vi "Centre Target.vi"(0 "Focus and Tracking":T4, 1 "Calibration":T5, 2 "System of Reference Interface":T3, 3 "Target":T2, 5 "error in (no error)":errorcluster, 9 "Refocus threshold":dbl=0.125) -> (13 "CFS":dbl, 14 "Target Coordinates [um]":T1, 15 "Optical Coordinates [um]":cluster{"X":dbl, "Y":dbl, "Z":dbl}, 16 "Need to refocus":bool, 17 "Scope Error":bool, 18 "Target OK":bool, 19 "error out":errorcluster)   [LabVIEW 2012, in "Targeting Unit.lvlib"]
uses:
  Targeting Unit.lvlib
  <vilib>/Analysis/Matrix/Datatypes/RealMatrix.ctl
  <vilib>/Analysis/Matrix/NI_Matrix.lvlib
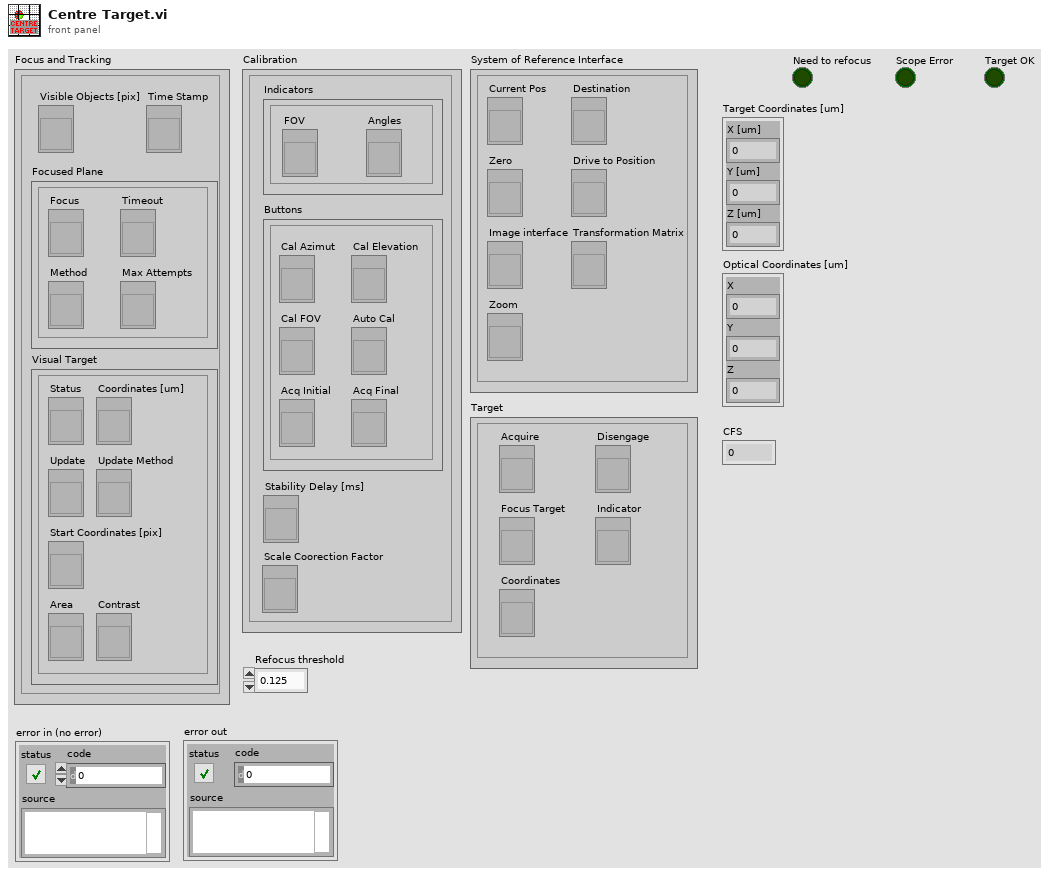
[diagram p1: front panel]
types:
  T1 = cluster{"X [um]":dbl, "Y [um]":dbl, "Z [um]":dbl}
  T2 = cluster{"Coordinates":refnum<vi>, "Acquire":refnum<vi>, "Disengage":refnum<vi>, "Indicator":refnum<vi>, "Focus Target":refnum<vi>}
  T3 = cluster{"Current Pos":refnum<vi>, "Image interface":refnum<vi>, "Transformation Matrix":refnum<vi>, "Zero":refnum<vi>, "Destination":refnum<vi>, "Drive to Position":refnum<vi>, "Zoom":refnum<vi>}
  T4 = cluster{"Focused Plane":cluster{"Focus":refnum<vi>, "Timeout":refnum<vi>, "Max Attempts":refnum<vi>, "Method":refnum<vi>}, "Time Stamp":refnum<vi>, "Visual Target":cluster{"Coordinates [um]":refnum<vi>, "Status":refnum<vi>, "Update":refnum<vi>, "Update Method":refnum<vi>, "Start Coordinates [pix]":refnum<vi>, "Area":refnum<vi>, "Contrast":refnum<vi>}, "Visible Objects [pix]":refnum<vi>}
  T5 = cluster{"Indicators":cluster{"FOV":refnum<vi>, "Angles":refnum<vi>}, "Buttons":cluster{"Cal FOV":refnum<vi>, "Cal Azimut":refnum<vi>, "Cal Elevation":refnum<vi>, "Auto Cal":refnum<vi>, "Acq Initial":refnum<vi>, "Acq Final":refnum<vi>}, "Stability Delay [ms]":refnum<vi>, "Scale Coorection Factor":refnum<vi>}
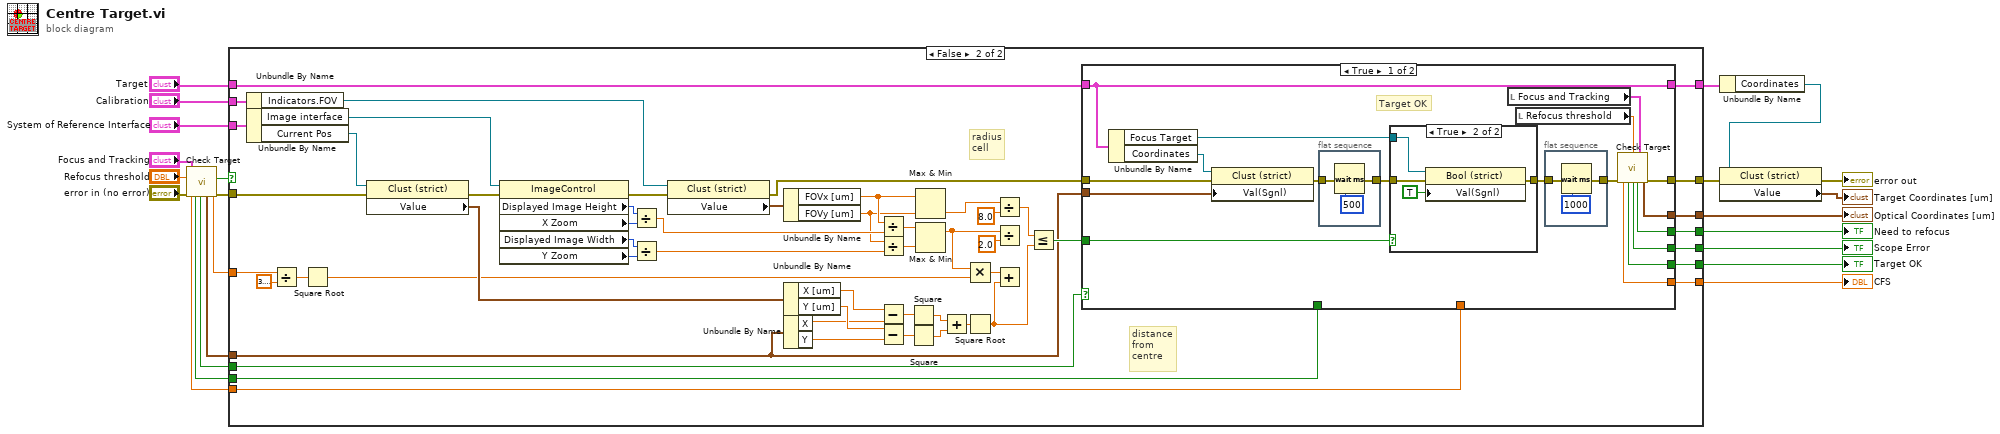
[diagram p0: block diagram]
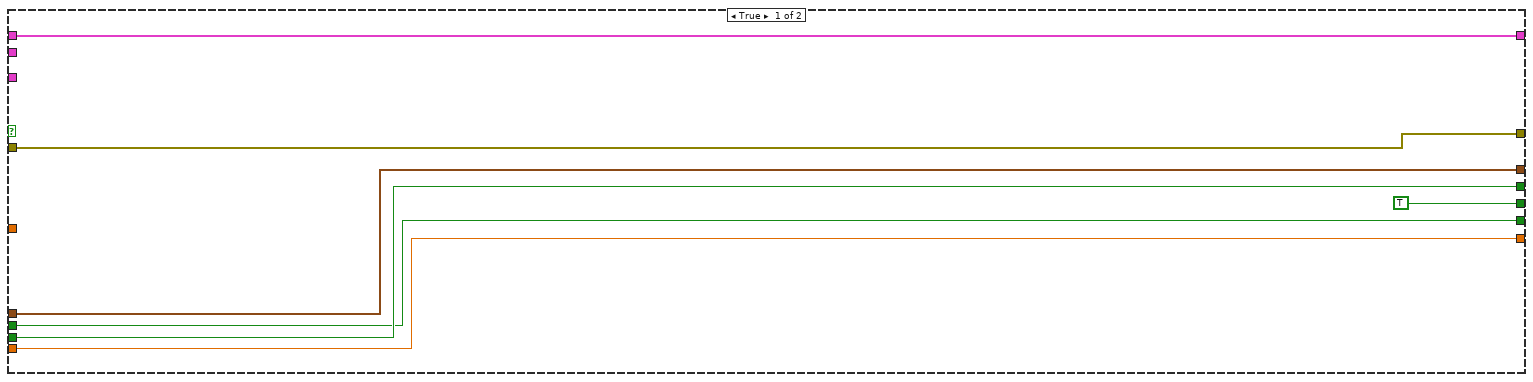
[diagram p2: hidden frame]
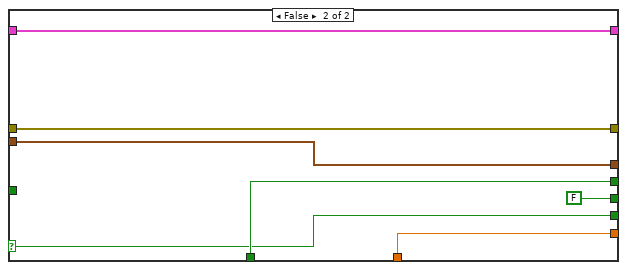
[diagram p4: hidden frame]
diagram:
  n1 = call "Check Target.vi"("Error In"="error in (no error)", "Refocus threshold"="Refocus threshold", "Focus and Tracking"="Focus and Tracking") -> ("Error out"=w16:errorcluster, "CFS"=w6:dbl, "Scope Error"=w14:bool, "Target OK"=w2:bool, "Optical Coordinates [um]"=w12:cluster{"X":dbl, "Y":dbl, "Z":dbl}, "Need to refocus"=w5:bool, "Area"=w1:dbl)  [unwired: 2 in]
  n2 = case shown="False" w14 {
    tunnel: "Calibration" -> [_ w74]
    tunnel: "System of Reference Interface" -> [_ w73]
    tunnel: [w27 w58] -> w20
    tunnel: w16 -> [w27 w43]
    tunnel: [TRUE ("Error") w50] -> w21
    tunnel: w12 -> [w29 w45]
    tunnel: "Target" -> [w28 w56]
    tunnel: [w29 w54] -> w9
    tunnel: [w28 w55] -> w8
    tunnel: [w25 w53] -> w7
    tunnel: w6 -> [w26 w52]
    tunnel: w5 -> [w25 w51]
    tunnel: [w24 w49] -> w3
    tunnel: [w26 w48] -> w4
    tunnel: w2 -> [w24 w47]
    tunnel: w1 -> [_ w44]
    frame True {
    }
    frame False {
      # "distance\nfrom\ncentre"
      # "radius\ncell"
      n3 = Unbundle By Name(w74) -> ("Indicators.FOV"=w75:refnum<vi>)
      n4 = Unbundle By Name(w73) -> ("Image interface"=w62:refnum<vi>, "Current Pos"=w68:refnum<vi>)
      n5 = Divide(x=w44, y=3.141592653589793) -> (x/y=w76:dbl)
      n6 = Square Root(x=w76) -> (sqrt(x)=w41:dbl)
      n7 = property class="Clust (strict)"(reference=w68, error in=w43) -> (error out=w42:errorcluster, "Value"=w77:T1)  [unwired: 1 out]
      n8 = property class="ImageControl"(reference=w62, error in=w42) -> (error out=w67:errorcluster, "Displayed Image Height"=w72:u32, "X Zoom"=w71:i32, "Displayed Image Width"=w70:u32, "Y Zoom"=w69:i32)  [unwired: 1 out]
      n9 = Divide(x=w72, y=w71) -> (x/y=w66:dbl)
      n10 = Divide(x=w70, y=w69) -> (x/y=w65:dbl)
      n11 = property class="Clust (strict)"(reference=w75, error in=w67) -> (error out=w57:errorcluster, "Value"=w84:cluster{"FOVx [um]":dbl, "FOVy [um]":dbl})  [unwired: 1 out]
      n12 = Unbundle By Name(w84) -> ("FOVx [um]"=w36:dbl, "FOVy [um]"=w35:dbl)
      n13 = Unbundle By Name(w77) -> ("X [um]"=w78:dbl, "Y [um]"=w81:dbl)
      n14 = Unbundle By Name(w45) -> ("X"=w79:dbl, "Y"=w80:dbl)
      n15 = Divide(x=w36, y=w66) -> (x/y=w64:dbl)
      n16 = Divide(x=w35, y=w65) -> (x/y=w63:dbl)
      n17 = Subtract(x=w78, y=w79) -> (x-y=w82:dbl)
      n18 = Subtract(x=w81, y=w80) -> (x-y=w83:dbl)
      n19 = Square(x=w82) -> (x^2=w61:dbl)
      n20 = Square(x=w83) -> (x^2=w60:dbl)
      n21 = Max & Min(x=w36, y=w35) -> (min(x,y)=w33:dbl)  [unwired: 1 out]
      n22 = Max & Min(x=w64, y=w63) -> (max(x,y)=w37:dbl)  [unwired: 1 out]
      n23 = Add(x=w61, y=w60) -> (x+y=w59:dbl)
      n24 = Multiply(x=w37, y=w41) -> (x*y=w39:dbl)
      n25 = Square Root(x=w59) -> (sqrt(x)=w31:dbl)
      n26 = Divide(x=w33, y=8.0) -> (x/y=w32:dbl)
      n27 = Divide(x=w37, y=2.0) -> ()  [unwired: 1 out]
      n28 = Add(x=w39, y=w31) -> ()  [unwired: 1 out]
      n29 = Less Or Equal?(x=w32, y=w31) -> (x <= y?=w46:bool)
      n30 = case shown="True" w47 {
        selector: w47 -> [_ w112]
        tunnel: [w96 w118] -> w58
        tunnel: w57 -> [w98 w118]
        tunnel: w45 -> [w99 w116]
        tunnel: w56 -> [w87 w117]
        tunnel: [w87 w117] -> w55
        tunnel: [w95 w116] -> w54
        tunnel: [w94 w113] -> w53
        tunnel: w52 -> [_ w115]
        tunnel: w51 -> [_ w113]
        tunnel: [w93 FALSE ("Scope Error")] -> w50
        tunnel: [w92 w112] -> w49
        tunnel: [w91 w115] -> w48
        tunnel: w46 -> [w90 _]
        frame True {
          # "Target OK"
          n31 = Unbundle By Name(w87) -> ("Focus Target"=w97:refnum<vi>, "Coordinates"=w100:refnum<vi>)
          n32 = property class="Clust (strict)"(reference=w100, error in=w98, "Val(Sgnl)"=w99) -> (error out=w102:errorcluster)  [unwired: 1 out]
          n33 = flat-sequence {
            tunnel: [w111] -> w101
            tunnel: w102 -> [w111]
            frame #0 {
              n34 = Wait (ms)(milliseconds to wait=u32 500) -> ()  [unwired: 1 out]
            }
          }
          n35 = case shown="True" w90 {
            tunnel: w101 -> [w105 w109]
            tunnel: w97 -> [_ w107]
            tunnel: [w105 w106] -> w86
            frame False {
            }
            frame True {
              n36 = property class="Bool (strict)"(reference=w107, error in=w109, "Val(Sgnl)"=TRUE ("Value (Signaling)")) -> (error out=w106:errorcluster)  [unwired: 1 out]
            }
          }
          n37 = local read "Focus and Tracking"() -> (w89:T4)
          n38 = local read "Refocus threshold"() -> (w88:dbl)
          n39 = flat-sequence {
            tunnel: [w104] -> w85
            tunnel: w86 -> [w104]
            frame #0 {
              n40 = Wait (ms)(milliseconds to wait=u32 1000) -> ()  [unwired: 1 out]
            }
          }
          n41 = call "Check Target.vi"("Error In"=w85, "Refocus threshold"=w88, "Focus and Tracking"=w89) -> ("Error out"=w96:errorcluster, "CFS"=w91:dbl, "Scope Error"=w93:bool, "Target OK"=w92:bool, "Optical Coordinates [um]"=w95:cluster{"X":dbl, "Y":dbl, "Z":dbl}, "Need to refocus"=w94:bool)  [unwired: 2 in, 1 out]
        }
        frame False {
        }
      }
    }
  }
  "Scope Error" <- w21
  "Need to refocus" <- w7
  "CFS" <- w4
  "Optical Coordinates [um]" <- w9
  "Target OK" <- w3
  n42 = Unbundle By Name(w8) -> ("Coordinates"=w18:refnum<vi>)
  n43 = property class="Clust (strict)"(reference=w18, error in=w20) -> (error out=→"error out":errorcluster, "Value"=→"Target Coordinates [um]":T1)  [unwired: 1 out]
